vi "arduino.vi"() -> ()   [LabVIEW 2013]
uses:
  <vilib>/LabVIEW Interface for Arduino/Type Defs/Board Type.ctl
  <vilib>/LabVIEW Interface for Arduino/Type Defs/Connection Type.ctl
  <vilib>/LabVIEW Interface for Arduino/Type Defs/Pin Mode.ctl
  <vilib>/LabVIEW Interface for Arduino/LabVIEW Interface for Arduino.lvlib
panel:
  in  "VISA resource":refnum<visa-resource-name>
  in  "ON":bool
  in  "Pin Mode (Input)":T1
  in  "Digital I/O Pin (0)":u8
  in  "Connection Type (USB/Serial)":T2
  in  "Board Type (Uno)":T3
  in  "Baud Rate (115200)":u32=115200
  in  "stop":bool
  # "UNIVERSIDAD DE CUNDINAMARCA\nINGENIERIA DE SISTEMAS\nELECTIVA PROFESIONAL IV\nANDY CAMARGO\nRAFAEL REYES\nSEMESTRE X\nEXTENCION CHIA"
  # "OFF"
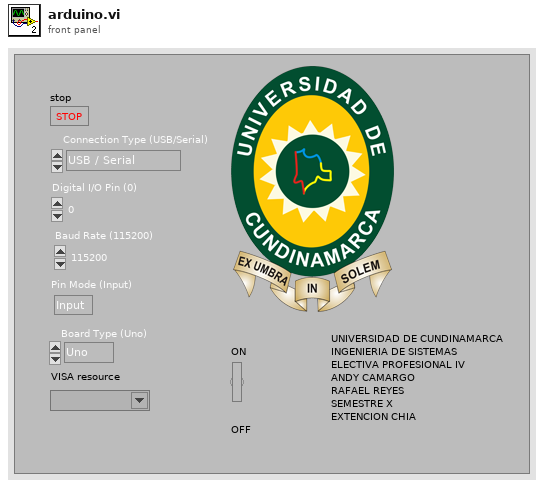
[diagram p1: front panel]
types:
  T1 = typedef "LabVIEW Interface for Arduino.lvlib/Pin Mode.ctl" = enum8{"Input", "Output"}
  T2 = typedef "LabVIEW Interface for Arduino.lvlib/Connection Type.ctl" = enum8{"USB / Serial", "XBEE", "BlueSmirf (Bluetooth)"}
  T3 = typedef "LabVIEW Interface for Arduino.lvlib/Board Type.ctl" = enum16{"Uno", "Dimuelanove w/Atmega 328", "Mega 2560"}
  T4 = typedef "LabVIEW Interface for Arduino.lvlib/Arduino Resource.ctl" = cluster{"VISA resource":refnum<visa-resource-name>, "Board Type":T3, "Connection Type":enum8{"USB / Serial"}, "Bytes Per Packet (15)":u8}
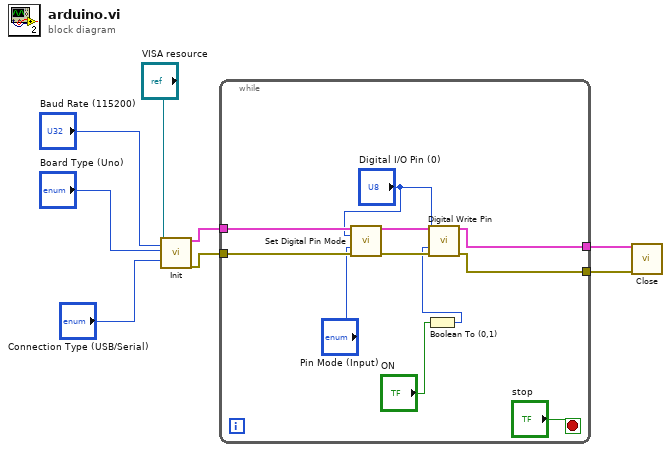
[diagram p0: block diagram]
diagram:
  n1 = call <vilib>:"Init.vi"("VISA resource"="VISA resource", "Baud Rate (115200)"="Baud Rate (115200)", "Board Type (Uno)"="Board Type (Uno)", "Connection Type (USB/Serial)"="Connection Type (USB/Serial)") -> ("Arduino Resource"=w8:T4, "error out"=w6:errorcluster)  [unwired: 14 in]
  n2 = while {
    tunnel: w8 -> [w18]
    tunnel: [w16] -> w7
    tunnel: w6 -> [w15]
    tunnel: [w13] -> w5
    stop <- "stop" stop-if-true
    n3 = call <vilib>:"Set Digital Pin Mode.vi"("Arduino Resource"=w18, "Digital I/O Pin"="Digital I/O Pin (0)", "Pin Mode (Input)"="Pin Mode (Input)", "error in"=w15) -> ("Arduino Resource"=w17:T4, "error out"=w14:errorcluster)  [unwired: 10 in]
    n4 = Boolean To (0,1)(Boolean="ON") -> (0, 1=w9:i16)
    n5 = call <vilib>:"Digital Write Pin.vi"("Arduino Resource"=w17, "Digital I/O Pin (0)"="Digital I/O Pin (0)", "Value (0)"=w9, "error in"=w14) -> ("Arduino Resource"=w16:T4, "error out"=w13:errorcluster)  [unwired: 10 in]
  }
  n6 = call <vilib>:"Close.vi"("Arduino Resource"=w7, "error in"=w5) -> ()  [unwired: 13 in, 1 out]
